vi "DequeueCmd.vi"(0 "cmdRef in":T1, 5 "timeout in ms (-1)":i32, 11 "error in (no error)":errorcluster) -> (4 "cmdRef out":T1, 6 "postdata":string, 10 "timed out?":bool, 15 "error out":errorcluster)   [LabVIEW 2017, in "vsws.lvlib"]
uses:
  vsws.lvlib
  cmdRef.ctl
  cmd.ctl
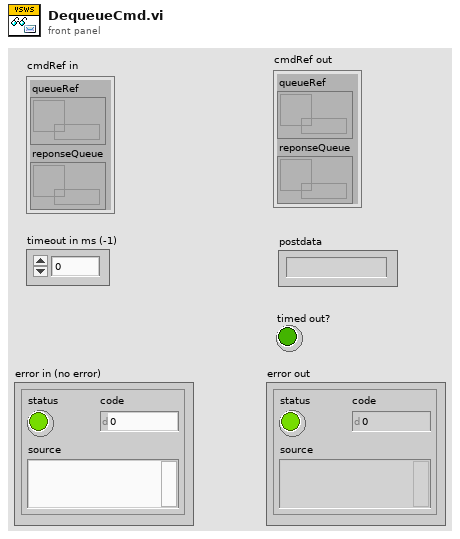
[diagram p1: front panel]
types:
  T1 = typedef "vsws.lvlib/cmdRef.ctl" = cluster{"queueRef":refnum<queue>, "reponseQueue":refnum<queue>}
  T2 = typedef "vsws.lvlib/cmd.ctl" = cluster{"postdata":string, "reponseQueue":refnum<queue>}
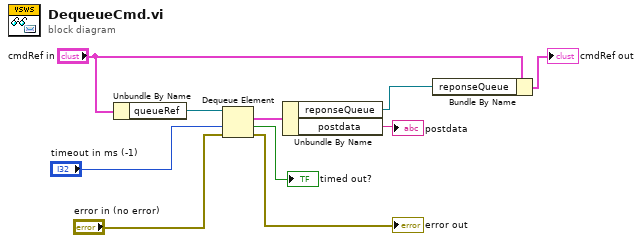
[diagram p0: block diagram]
diagram:
  n1 = Unbundle By Name("cmdRef in") -> ("queueRef"=w10:refnum<queue>)
  n2 = Dequeue Element(queue=w10, timeout in ms (-1)="timeout in ms (-1)", error in (no error)="error in (no error)") -> (element=w4:T2, timed out?=→"timed out?":bool, error out=→"error out":errorcluster)  [unwired: 1 out]
  n3 = Unbundle By Name(w4) -> ("reponseQueue"=w2:refnum<queue>, "postdata"=→"postdata":string)
  n4 = Bundle By Name(cluster="cmdRef in", "reponseQueue"=w2) -> (→"cmdRef out":T1)
